vi "Lamp Power.vi"(8 "error in (no error)":errorcluster, 10 "On/Off":enum16{"Off", "On"}(ring), 11 "Neph in":refnum<class "Nephelometer.lvclass">) -> (0 "error out":errorcluster, 3 "Neph out":refnum<class "Nephelometer.lvclass">)   [LabVIEW 2014, in "Nephelometer.lvclass"]
uses:
  Nephelometer.lvclass
  Nephelometer.lvclass/Nephelometer.ctl
  Accessors/Read Session Handle.vi
  Reusable/Session APIs/Serial/Public/Get Data/Get String.vi
  <userlib>/_Session Fwk/Session - Root.lvclass
  Reusable/Session APIs/Text Communication/Text Device Session.lvclass
panel:
  out "Read - Asynchronous":string
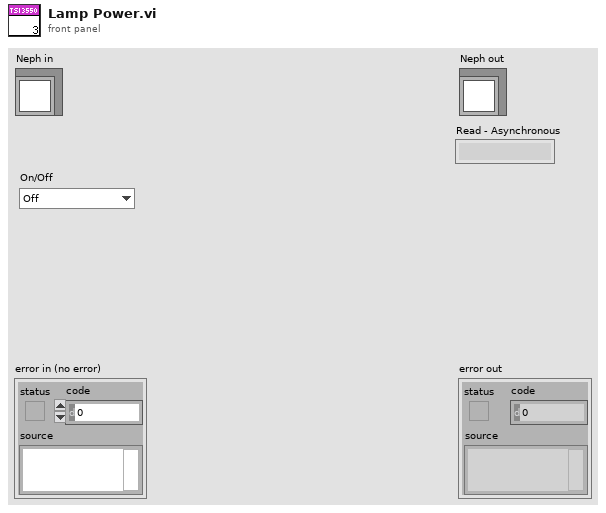
[diagram p1: front panel]
types:
  T1 = typedef "Session - Root.lvclass/Session Handle.ctl" = refnum<data-value>
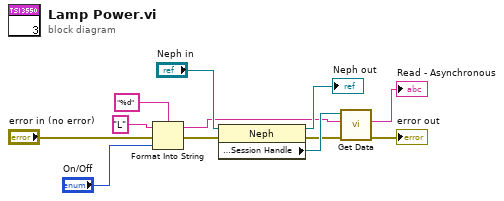
[diagram p0: block diagram]
diagram:
  n1 = Format Into String(format string="%d", initial string="L", error in="error in (no error)", "On/Off") -> (resulting string=w4:string, error out=w8:errorcluster)
  n2 = property class="Neph"(reference="Neph in", error in=w8) -> (reference out=→"Neph out":refnum<class "Nephelometer.lvclass">, error out=w2:errorcluster, "Accessors:Session Handle"=w5:T1)
  n3 = call-poly "Get Data.vi"("error in"=w2, "CMD"=w4, "handle in"=w5) -> ("error out"=→"error out":errorcluster, "DataOut"=→"Read - Asynchronous":string)  [unwired: 6 in, 1 out]
